vi "1_Waveform_Signal_Regression(Training).vi"() -> ()   [LabVIEW 2020]
uses:
  <vilib>/Ngene/DeepLTK/Toolkit/NN_Train/Controls/NN_LR_Policy_Cfg.ctl
  <vilib>/Ngene/DeepLTK/Toolkit/NN_Train/Controls/NN_LR_Policy_Type.ctl
  <vilib>/Ngene/DeepLTK/Toolkit/NN_Train/Controls/NN_Train_Session_Data.ctl
  <vilib>/Ngene/DeepLTK/Toolkit/NN_Train/Controls/NN_Train_Params.ctl
  <vilib>/Ngene/DeepLTK/Toolkit/NN_Train/Controls/NN_Train_Optimizer.ctl
  <vilib>/Ngene/DeepLTK/Toolkit/NN_Train/Controls/NN_Train_Data_Sampling.ctl
  <vilib>/Ngene/DeepLTK/Toolkit/NN_Network/Controls/NN_Device.ctl
  <vilib>/Ngene/DeepLTK/Toolkit/NN_Layers/Layers/Input/Controls/NN_Layer_Config(Input1D).ctl
  <vilib>/Ngene/DeepLTK/Toolkit/NN_Layers/Layers/FC/Controls/NN_Layer_Config(FC).ctl
  <vilib>/Ngene/DeepLTK/Toolkit/NN_Activations/Controls/NN_Activation_Type.ctl
  <vilib>/Ngene/DeepLTK/Toolkit/NN_Layers/Controls/NN_Layer_Init_Params.ctl
  <vilib>/Ngene/DeepLTK/Toolkit/NN_Layers/Controls/NN_Layer_Weight_Init_Type.ctl
  <vilib>/Ngene/DeepLTK/Toolkit/NN_Network/Controls/NN_Save_Before_Destroy_Options.ctl
  <vilib>/Ngene/DeepLTK/Toolkit/NN_Layers/Layers/Input/NN_Layer_Create(Input1D).vi
  <vilib>/Ngene/DeepLTK/Toolkit/NN_Layers/Layers/FC/NN_Layer_Create(FC).vi
  <vilib>/Ngene/DeepLTK/Toolkit/NN_Train/Loss_Functions/NN_Set_Loss(MSE).vi
  <vilib>/Ngene/DeepLTK/Toolkit/NN_Network/subVIs/NN_Predict/NN_Predict(In1D_Out1D).vi
  <vilib>/Ngene/DeepLTK/Toolkit/NN_Train/Eval_Loss/NN_Eval_Test_Error_Loss/NN_Eval(In1D_Out1D).vi
  <vilib>/Ngene/DeepLTK/Toolkit/Deep_Learning_Toolkit_by_Ngene.lvlib
  <vilib>/ptbypt/NI_PtbyPt.lvlib
panel:
  out "Training Loss":sgl=30.107077 format="%#.6g"
  in  "Eval":bool
  out "Loss Graphs":cluster{"mean":dbl, "mean":dbl}(graph)={"mean"=10.700733497142792, "mean"=0.33381223678588867}
  in  "NN_Device":T1=enum."GPU"
  out "Test Loss":sgl=0.33381224 format="%#.6g"
  in  "Stop Training":bool
  in  "NN_Train_Params":T2={"Optimizer"=enum."Adam", "Beta_1"=0.9, "Beta_2"=0.999, "Weight Decay(L1)"=1e-07, "Weight Decay(L2)"=1e-07, "Data_Sampling"=enum."Random"}
  out "Session Data":T5={"Epochs"=22.1088, "Tot_Iter"=13818, "LR"=0.0025, "LR_iter"=13819} {"LR" format="%#_3g"}
  in  "LR Update Policy":T6={"Policy_Type"=enum."Step", "LR0"=0.010000000000000002, "k"=10.0, "WarmUp_Policy"=enum."Ramp", "WarmUp_Iter"=1000, "WarmUp_Ratio"=100.0} {"WarmUp_Ratio" min=1; "WarmUp_Iter" min=1; "LR0" format="%.7f"}
  # "Overview: This example demonstrating the usage of Deep Learning Toolkit for solving  waveform signal regression problem.\nRequirements: Deep Learning Toolkit for LabVIEW\nInstructions:\n1.  Run the VI with current configuration of the training parameters and Learning Rate update policy.\n2. Observe how the training loss is decreasing.\n3. Press the \"Stop Training\" when the loss is not decreasing any more."
  # "Waveform Signal Regression (Frequency Prediction) - Training"
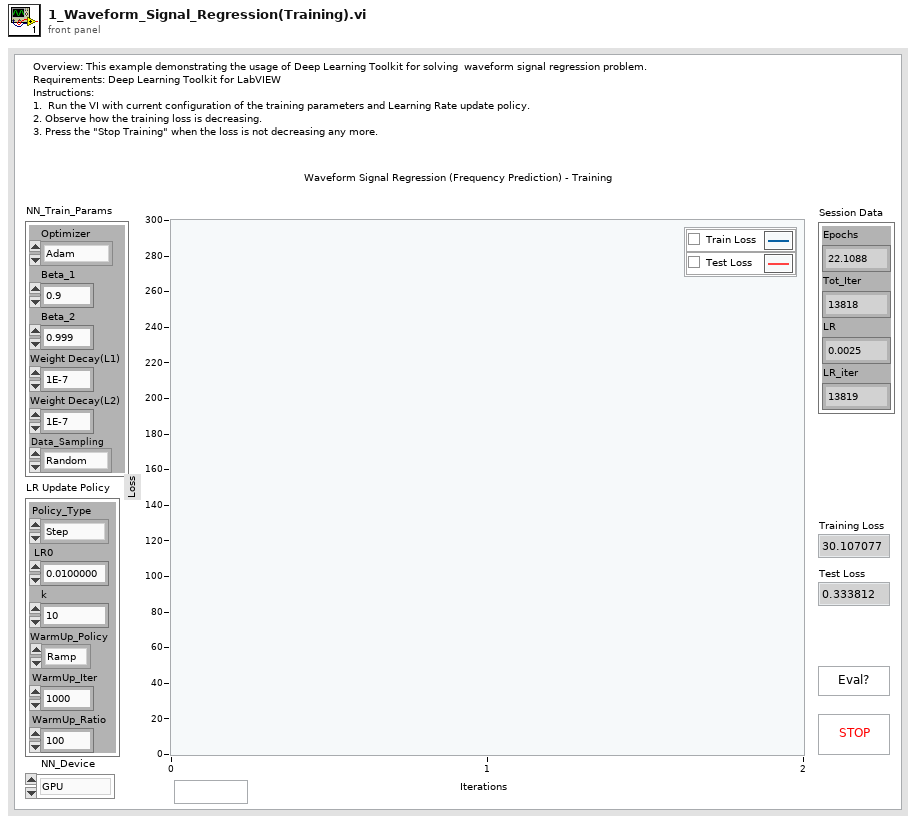
[diagram p1: front panel]
types:
  T1 = typedef "Deep_Learning_Toolkit_by_Ngene.lvlib/NN_Device.ctl" = enum16{"CPU", "GPU"}
  T2 = typedef "Deep_Learning_Toolkit_by_Ngene.lvlib/NN_Train_Params.ctl" = cluster{"Optimizer":T3, "Beta_1":sgl, "Beta_2":sgl, "Weight Decay(L1)":sgl, "Weight Decay(L2)":sgl, "Data_Sampling":T4}
  T3 = typedef "Deep_Learning_Toolkit_by_Ngene.lvlib/NN_Train_Optimizer.ctl" = enum16{"SGD", "Adam", "Adagrad", "Adadelta", "RMSProp", "Nesterov"}
  T4 = typedef "Deep_Learning_Toolkit_by_Ngene.lvlib/NN_Train_Data_Sampling.ctl" = enum16{"Random", "Sequential"}
  T5 = typedef "Deep_Learning_Toolkit_by_Ngene.lvlib/NN_Train_Session_Data.ctl" = cluster{"Epochs":sgl, "Tot_Iter":i32, "LR":sgl, "LR_iter":i32}
  T6 = typedef "Deep_Learning_Toolkit_by_Ngene.lvlib/NN_LR_Policy_Cfg.ctl" = cluster{"Policy_Type":T7, "LR0":dbl, "k":sgl, "WarmUp_Policy":enum16{"Step", "Ramp"}, "WarmUp_Iter":i32, "WarmUp_Ratio":sgl}
  T7 = typedef "Deep_Learning_Toolkit_by_Ngene.lvlib/NN_LR_Policy_Type.ctl" = enum16{"Manual", "Step", "Exp", "1/t"}
  T8 = typedef "Deep_Learning_Toolkit_by_Ngene.lvlib/NN_Save_Before_Destroy_Options.ctl" = cluster{"CFG?":bool, "Weights?":bool, "Render?":bool}
  T9 = typedef "Deep_Learning_Toolkit_by_Ngene.lvlib/NN_Layer_Config(FC).ctl" = cluster{"Name":string, "Size":i32, "BN":bool, "Activation":T10, "Init_Params":T11, "Custom_Params":string}
  T10 = typedef "Deep_Learning_Toolkit_by_Ngene.lvlib/NN_Activation_Type.ctl" = enum16{"Sigmoid", "ReLU", "LReLU", "ReLU6", "tanh", "Swish", "Mish", "None"}
  T11 = typedef "Deep_Learning_Toolkit_by_Ngene.lvlib/NN_Layer_Init_Params.ctl" = cluster{"Init_Type":T12, "Value":sgl}
  T12 = typedef "Deep_Learning_Toolkit_by_Ngene.lvlib/NN_Layer_Weight_Init_Type.ctl" = enum16{"Const", "Uniform", "Gaussian", "Xavier"}
  T13 = typedef "Deep_Learning_Toolkit_by_Ngene.lvlib/NN_Layer_Config(Input1D).ctl" = cluster{"Name":string, "Size":i32}
  T14 = typedef "Deep_Learning_Toolkit_by_Ngene.lvlib/NN_DataSets_All(In1D_Out1D).ctl" = cluster{"Train":T15, "Validation":T15, "Test":T15}
  T15 = typedef "Deep_Learning_Toolkit_by_Ngene.lvlib/NN_DataSet(In1D_Out1D).ctl" = cluster{"Inputs Ref.":T16, "Outputs Ref.":T16, "Dims_In":i32, "Dataset_Size":i32, "Outputs_idx Ref.":T17, "Dims_Out":i32, "Labels":string[], "File Paths":path[]}
  T16 = typedef "Deep_Learning_Toolkit_by_Ngene.lvlib/NN_Data_ref(2D_SGL).ctl" = refnum<data-value>
  T17 = typedef "Deep_Learning_Toolkit_by_Ngene.lvlib/NN_Data_ref(1D_I32).ctl" = refnum<data-value>
  T18 = typedef "Deep_Learning_Toolkit_by_Ngene.lvlib/NN.ctl" = cluster{"Name":string, "No of Layers":i32, "mBatch":i32, "Layers":T19[], "Dimty":T20, "Dims_In":T21, "Dims_Out":T21, "Working_Dir":path, "Train?":bool, "Train_Params":T2, "LR_Update_Policy":T6, "Session Data":T5, "Ground_truth":T22, "NNg_hdls":T23, "NN_Device":T1, "GPU Id":i32, "Labels":string[], "Receptive Field":T24[], "Loss_Type":T25, "Loss_Cfg_Prms":variant}
  T19 = typedef "Deep_Learning_Toolkit_by_Ngene.lvlib/NN_Layer_ref.ctl" = refnum<data-value>
  T20 = typedef "Deep_Learning_Toolkit_by_Ngene.lvlib/NN_In_Out_Dim-ty.ctl" = enum8{"In1D_Out1D", "In3D_Out1D", "In3D_Out3D", "In3D_OutBBox"}
  T21 = typedef "Deep_Learning_Toolkit_by_Ngene.lvlib/NN_Dims(C,H,W).ctl" = cluster{"C":i32, "H":i32, "W":i32}
  T22 = typedef "Deep_Learning_Toolkit_by_Ngene.lvlib/NN_Ground_truth.ctl" = cluster{"Y":variant, "Y_idx":T17}
  T23 = typedef "Deep_Learning_Toolkit_by_Ngene.lvlib/nng_cuda_handles.ctl" = cluster{"cudnn":u64, "cublas":u64, "stream":u64, "curand":u64}
  T24 = typedef "Deep_Learning_Toolkit_by_Ngene.lvlib/NN_Dims(V,H).ctl" = cluster{"V":i32, "H":i32}
  T25 = typedef "Deep_Learning_Toolkit_by_Ngene.lvlib/NN_Loss_Type.ctl" = enum16{"None", "MSE", "CrossEntropy", "YOLO_v2"}
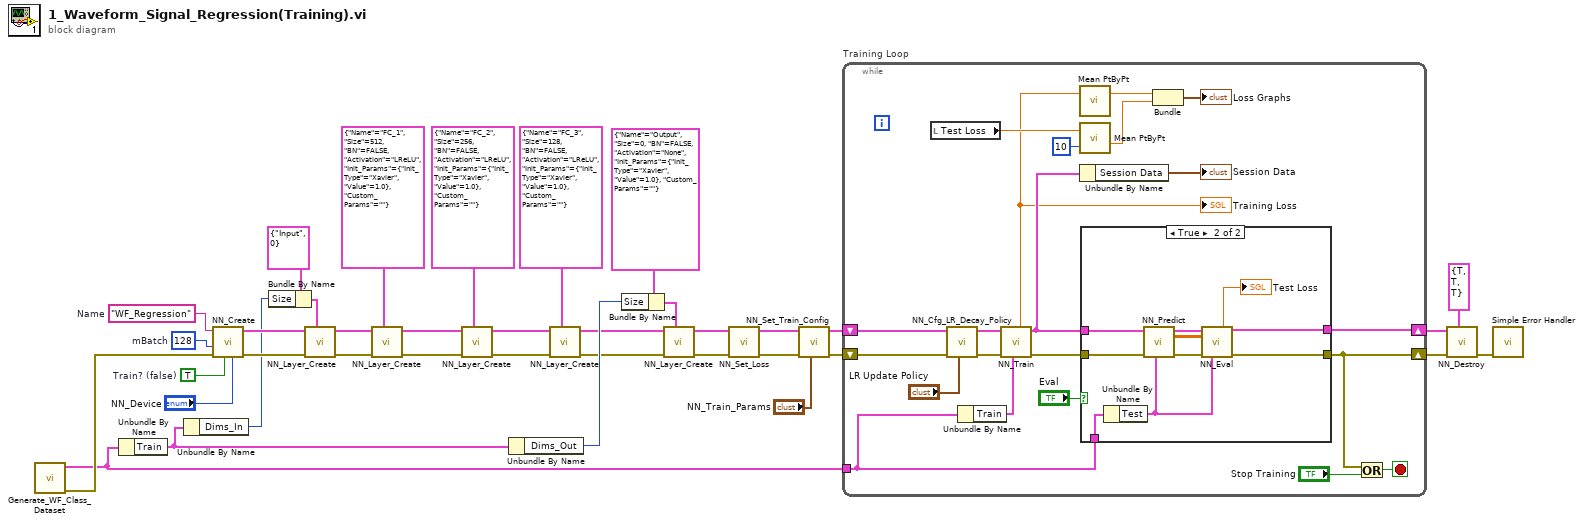
[diagram p0: block diagram]
diagram:
  w18 = "WF_Regression"  # Name
  w19 = 128  # mBatch
  w20 = TRUE  # Train? (false)
  n1 = call "Generate_WF_Class_Dataset.vi"() -> ("error out"=w29:errorcluster, "DataSets_All(In1D_Out1D)"=w3:T14)  [unwired: 10 in]
  n2 = Unbundle By Name(w3) -> ("Train"=w1:T15)
  n3 = Unbundle By Name(w1) -> ("Dims_In"=w27:i32)
  n4 = call <vilib>:"NN_Create.vi"("NN_Device"="NN_Device", "Train? (false)"=w20, "error in (no error)"=w29, "mBatch (1)"=w19, "Name"=w18) -> ("error out"=w36:errorcluster, "NN out"=w37:T18)  [unwired: 5 in]
  n5 = Bundle By Name(cluster=T13 {"Name"="Input", "Size"=0} ("Input1D_Cfg"), "Size"=w27) -> (w28:T13)
  n6 = call-poly <vilib>:"NN_Layer_Create.vi"("Input1D_Cfg"=w28, "error in (no error)"=w36, "NN in"=w37) -> ("error out"=w23:errorcluster, "NN out"=w24:T18)  [unwired: 6 in, 1 out]
  n7 = call-poly <vilib>:"NN_Layer_Create.vi"("FC_Cfg"=T9 {"Name"="FC_1", "Size"=512, "BN"=FALSE, "Activation"=enum."LReLU", "Init_Params"={"Init_Type"=enum."Xavier", "Value"=1.0}, "Custom_Params"=""} ("FC_Cfg_1"), "error in (no error)"=w23, "NN in"=w24) -> ("error out"=w12:errorcluster, "NN out"=w13:T18)  [unwired: 6 in, 1 out]
  n8 = call-poly <vilib>:"NN_Layer_Create.vi"("FC_Cfg"=T9 {"Name"="FC_2", "Size"=256, "BN"=FALSE, "Activation"=enum."LReLU", "Init_Params"={"Init_Type"=enum."Xavier", "Value"=1.0}, "Custom_Params"=""} ("FC_Cfg_1"), "error in (no error)"=w12, "NN in"=w13) -> ("error out"=w8:errorcluster, "NN out"=w9:T18)  [unwired: 6 in, 1 out]
  n9 = Unbundle By Name(w1) -> ("Dims_Out"=w25:i32)
  n10 = call-poly <vilib>:"NN_Layer_Create.vi"("FC_Cfg"=T9 {"Name"="FC_3", "Size"=128, "BN"=FALSE, "Activation"=enum."LReLU", "Init_Params"={"Init_Type"=enum."Xavier", "Value"=1.0}, "Custom_Params"=""} ("FC_Cfg_1"), "error in (no error)"=w8, "NN in"=w9) -> ("error out"=w6:errorcluster, "NN out"=w7:T18)  [unwired: 6 in, 1 out]
  n11 = Bundle By Name(cluster=T9 {"Name"="Output", "Size"=0, "BN"=FALSE, "Activation"=enum."None", "Init_Params"={"Init_Type"=enum."Xavier", "Value"=1.0}, "Custom_Params"=""} ("FC_Cfg_1"), "Size"=w25) -> (w26:T9)
  n12 = call-poly <vilib>:"NN_Layer_Create.vi"("FC_Cfg"=w26, "error in (no error)"=w6, "NN in"=w7) -> ("error out"=w32:errorcluster, "NN out"=w33:T18)  [unwired: 6 in, 1 out]
  n13 = call-poly <vilib>:"NN_Set_Loss.vi"("error in (no error)"=w32, "NN in"=w33) -> ("error out"=w15:errorcluster, "NN out"=w16:T18)  [unwired: 8 in]
  n14 = call <vilib>:"NN_Set_Train_Config.vi"("NN_Train_Params"="NN_Train_Params", "error in (no error)"=w15, "NN in"=w16) -> ("error out"=w21:errorcluster, "NN out"=w22:T18)  [unwired: 7 in]
  n15 = while "Training Loop" {
    shift-right: [w43] -> w4
    shift-left: w21 -> [w53]
    shift-right: [w49] -> w5
    shift-left: w22 -> [w56]
    tunnel: w3 -> [w39]
    stop <- w44 stop-if-true
    n16 = local read "Test Loss"() -> (w47:sgl)
    n17 = call <vilib>:"NN_Cfg_LR_Decay_Policy.vi"("LR_Decay_Params"="LR Update Policy", "error in (no error)"=w53, "NN in"=w56) -> ("error out"=w54:errorcluster, "NN out"=w55:T18)  [unwired: 7 in]
    n18 = Unbundle By Name(w39) -> ("Train"=w38:T15)
    n19 = call <vilib>:"NN_Train.vi"("Train Dataset"=w38, "error in (no error)"=w54, "NN in"=w55) -> ("error out"=w50:errorcluster, "NN out"=w51:T18, "Loss"=w45:sgl)  [unwired: 5 in, 1 out]
    "Training Loss" <- w45
    n20 = call <vilib>:"Mean PtByPt.vi"("x"=w45) -> ("mean"=w41:dbl)  [unwired: 3 in, 1 out]
    n21 = call <vilib>:"Mean PtByPt.vi"("x"=w47, "sample length"=10) -> ("mean"=w42:dbl)  [unwired: 2 in, 1 out]
    n22 = Unbundle By Name(w51) -> ("Session Data"=→"Session Data":T5)
    n23 = case shown="True" "Eval" {
      tunnel: w51 -> [w60 w69]
      tunnel: w50 -> [w59 w68]
      tunnel: [w60 w67] -> w49
      tunnel: [w59 w63] -> w43
      tunnel: w39 -> [_ w62]
      frame False {
      }
      frame True {
        n24 = Unbundle By Name(w62) -> ("Test"=w61:T15)
        n25 = call-poly <vilib>:"NN_Predict.vi"("Dataset"=w61, "error in (no error)"=w68, "NN in"=w69) -> ("error out"=w70:errorcluster, "Predictions"=w64:sgl[][], "NN out"=w65:T18)  [unwired: 6 in]
        n26 = call-poly <vilib>:"NN_Eval.vi"("NN in"=w65, "Predictions"=w64, "error in (no error)"=w70, "Dataset"=w61) -> ("Loss"=→"Test Loss":sgl, "NN out"=w67:T18, "error out"=w63:errorcluster)  [unwired: 7 in, 2 out]
      }
    }
    n27 = Bundle("mean"=w41, "mean"=w42) -> (→"Loss Graphs":cluster{"mean":dbl, "mean":dbl})  [unwired: 1 in]
    n28 = Or(x=w43, y="Stop Training") -> (x .or. y?=w44:bool)
  }
  n29 = call <vilib>:"NN_Destroy.vi"("Save (T, T, T)"=T8 {"CFG?"=TRUE, "Weights?"=TRUE, "Render?"=TRUE}, "error in (no error)"=w4, "NN in"=w5) -> ("error out"=w31:errorcluster)  [unwired: 8 in]
  n30 = call <vilib>:"Simple Error Handler.vi"("error in (no error)"=w31) -> ()  [unwired: 4 in, 5 out]
